vi "Buneman Frequency Estimator.vi"(0 "X":dbl[](array[numeric])) -> (1 "beta":dbl format="%.2f", 2 "error":i32)   [LabVIEW 2020, in "NI_Gmath.lvlib"]
doc: "Estimates the frequency of a given sine wave of unknown frequency using the Buneman formula."
uses:
  NI_Gmath.lvlib
  Real FFT.vi
  NI_AALPro.lvlib
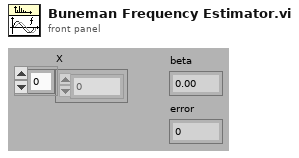
[diagram p1: front panel]
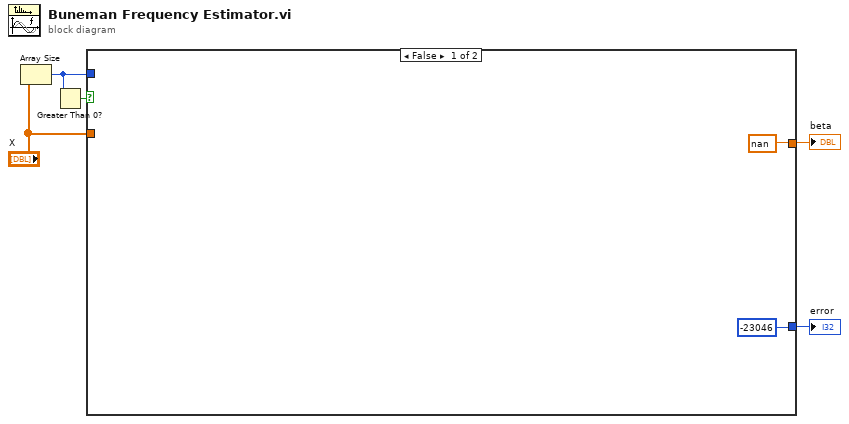
[diagram p0: block diagram]
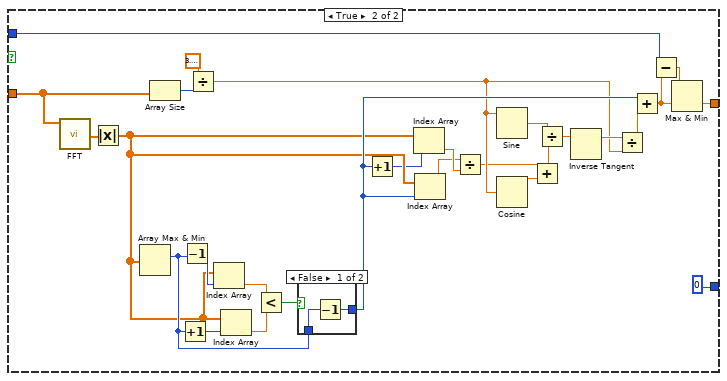
[diagram p2: hidden frame]
diagram:
  n1 = Array Size(array="X") -> (size(s)=w1:i32)
  n2 = Greater Than 0?(x=w1) -> (x > 0?=w2:bool)
  n3 = case shown="False" w2 {
    tunnel: "X" -> [_ w34]
    tunnel: [nan w11] -> w5
    tunnel: [-23046 0] -> w3
    tunnel: w1 -> [_ w10]
    frame False {
    }
    frame True {
      n4 = call-poly "FFT.vi"("X"=w34) -> ("FFT {X}"=w25:cdb[])  [unwired: 9 in, 1 out]
      n5 = Absolute Value(x=w25) -> (abs(x)=w26:dbl[])
      n6 = Array Max & Min(array=w26) -> (max index (indices)=w33:i32)  [unwired: 3 out]
      n7 = Array Size(array=w34) -> (size(s)=w35:i32)
      n8 = Increment(x=w33) -> (x+1=w28:i32)
      n9 = Decrement(x=w33) -> (x-1=w27:i32)
      n10 = Divide(x=3.141592653589793, y=w35) -> (x/y=w22:dbl)
      n11 = Index Array(array=w26, index=w27) -> (element=w29:dbl)
      n12 = Index Array(array=w26, index=w28) -> (element=w30:dbl)
      n13 = Less?(x=w29, y=w30) -> (x < y?=w31:bool)
      n14 = case shown="False" w31 {
        tunnel: w33 -> [w37 w38]
        tunnel: [w36 w38] -> w32
        frame False {
          n15 = Decrement(x=w37) -> (x-1=w36:i32)
        }
        frame True {
        }
      }
      n16 = Increment(x=w32) -> (x+1=w13:i32)
      n17 = Index Array(array=w26, index=w13) -> (element=w15:dbl)
      n18 = Index Array(array=w26, index=w32) -> (element=w14:dbl)
      n19 = Divide(x=w14, y=w15) -> (x/y=w17:dbl)
      n20 = Sine(x=w22) -> (sin(x)=w19:dbl)
      n21 = Cosine(x=w22) -> (cos(x)=w18:dbl)
      n22 = Add(x=w17, y=w18) -> (x+y=w20:dbl)
      n23 = Divide(x=w19, y=w20) -> (x/y=w21:dbl)
      n24 = Inverse Tangent(1:w21) -> (0:w23:dbl)
      n25 = Divide(x=w23, y=w22) -> (x/y=w24:dbl)
      n26 = Add(x=w32, y=w24) -> (x+y=w9:dbl)
      n27 = Subtract(x=w10, y=w9) -> (x-y=w8:dbl)
      n28 = Max & Min(x=w8, y=w9) -> (min(x,y)=w11:dbl)  [unwired: 1 out]
    }
  }
  "beta" <- w5
  "error" <- w3
